vi "Brookfield_Read_StandaloneMode.vi"() -> ()   [LabVIEW 2019]
uses:
  <vilib>/Instr/_visa.llb/VISA Configure Serial Port (Instr).vi
panel:
  out "Read Buffer (real time)":string
  out "Concatenated String":string
  # "PCProgON\nStandalone Mode"
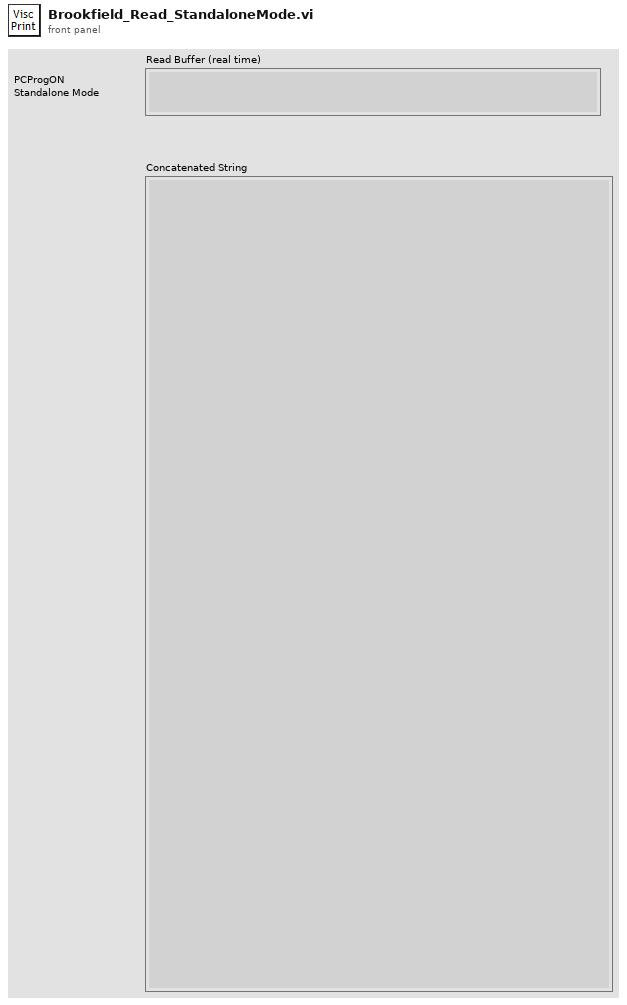
[diagram p1: front panel]
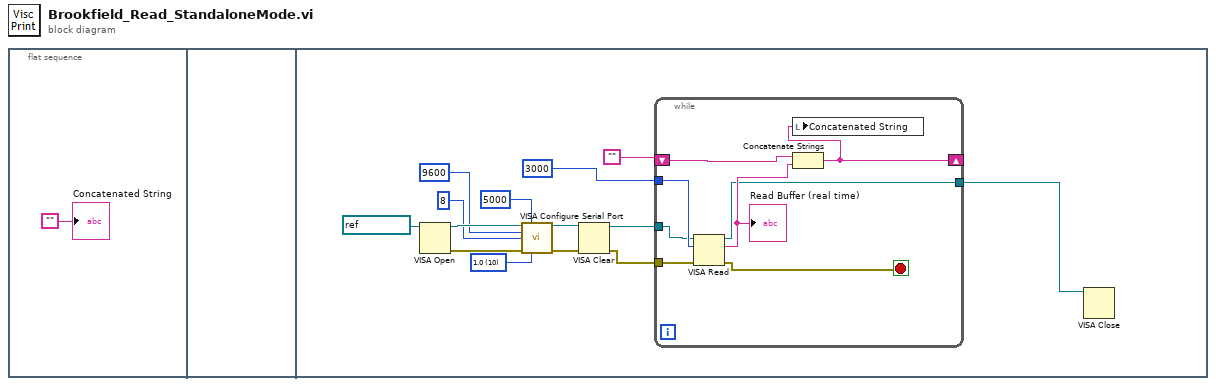
[diagram p0: block diagram]
diagram:
  n1 = flat-sequence {
    frame #0 {
      "Concatenated String" <- ""
    }
    frame #1 {
    }
    frame #2 {
      w8 = u16 10 items=["1.0"=10, "1.5"=15, "2.0"=20] ("stop bits (10: 1 bit)")
      n2 = VISA Open(VISA resource name=refnum<visa-resource-name> "COM10" ("Conductivity Port")) -> (VISA resource name=w12:refnum<visa-resource-name>, error out=w14:errorcluster)  [unwired: 4 in]
      n3 = call-poly "VISA Configure Serial Port"("VISA resource name"=w12, "timeout (10sec)"=u32 5000, "baud rate (9600)"=u32 9600, "data bits (8)"=u16 8, "error in (no error)"=w14, "stop bits (10: 1 bit)"=w8) -> ("VISA resource name out"=w5:refnum<visa-resource-name>, "error out"=w6:errorcluster)  [unwired: 8 in]
      n4 = VISA Clear(VISA resource name=w5, error in (no error)=w6) -> (VISA resource name out=w3:refnum<visa-resource-name>, error out=w4:errorcluster)
      n5 = while {
        tunnel: w4 -> [w23]
        tunnel: u32 3000 ("return count") -> [w22]
        tunnel: [w20] -> w15
        tunnel: w3 -> [w19]
        shift-right: [w17] -> _
        shift-left: "" -> [w18]
        stop <- w16 stop-if-true
        n6 = VISA Read(VISA resource name=w19, byte count=w22, error in (no error)=w23) -> (VISA resource name out=w20:refnum<visa-resource-name>, read buffer=w21:string, error out=w16:errorcluster)  [unwired: 1 out]
        "Read Buffer (real time)" <- w21
        n7 = Concatenate Strings(w18, w21) -> (w17:string)
        n8 = local write "Concatenated String"(w17) -> ()
      }
      n9 = VISA Close(VISA resource name=w15) -> ()  [unwired: 1 in, 1 out]
    }
  }
